vi "Detect Pulses in File.vi"(8 "Delay":dbl=0.013735 format="%#_6p", 9 "Channel name":string="CH0", 10 "I-V parameters":T1={"Start magnitude"=0.01, "Magnitude increment"=0.001, "Number of pulses"=8, "Baseline length"=480, "Ramp length"=32, "Top  length"=480, "Threshold "=1e-05, "Processing delay"=25, "Valhalla range"=0.001, "Interpolation"=64} {"Valhalla range" format="%#_6pA"; "Processing delay" format="%dpts"; "Threshold" format="%#_6pV"; "Top  length" format="%dpts"; "Ramp length" format="%dpts"; "Baseline length" format="%dpts"; "Magnitude increment" format="%#_6pA"; "Start magnitude" format="%#_6pA"}, 11 "File Path":path) -> (0 "Avg signal minus\nAvg background":dbl[](graph), 1 "Pulse indices out":T2[](array[typedef]), 2 "data":waveform(dbl))   [LabVIEW 2016]
uses:
  Pulse indexies.ctl
  I-V parameters.ctl
panel:
  in  "Skip 1st #points":i32=124993
  out "Waveform Graph 2":dbl[][](graph)
  out "Waveform Graph":dbl[][](graph)
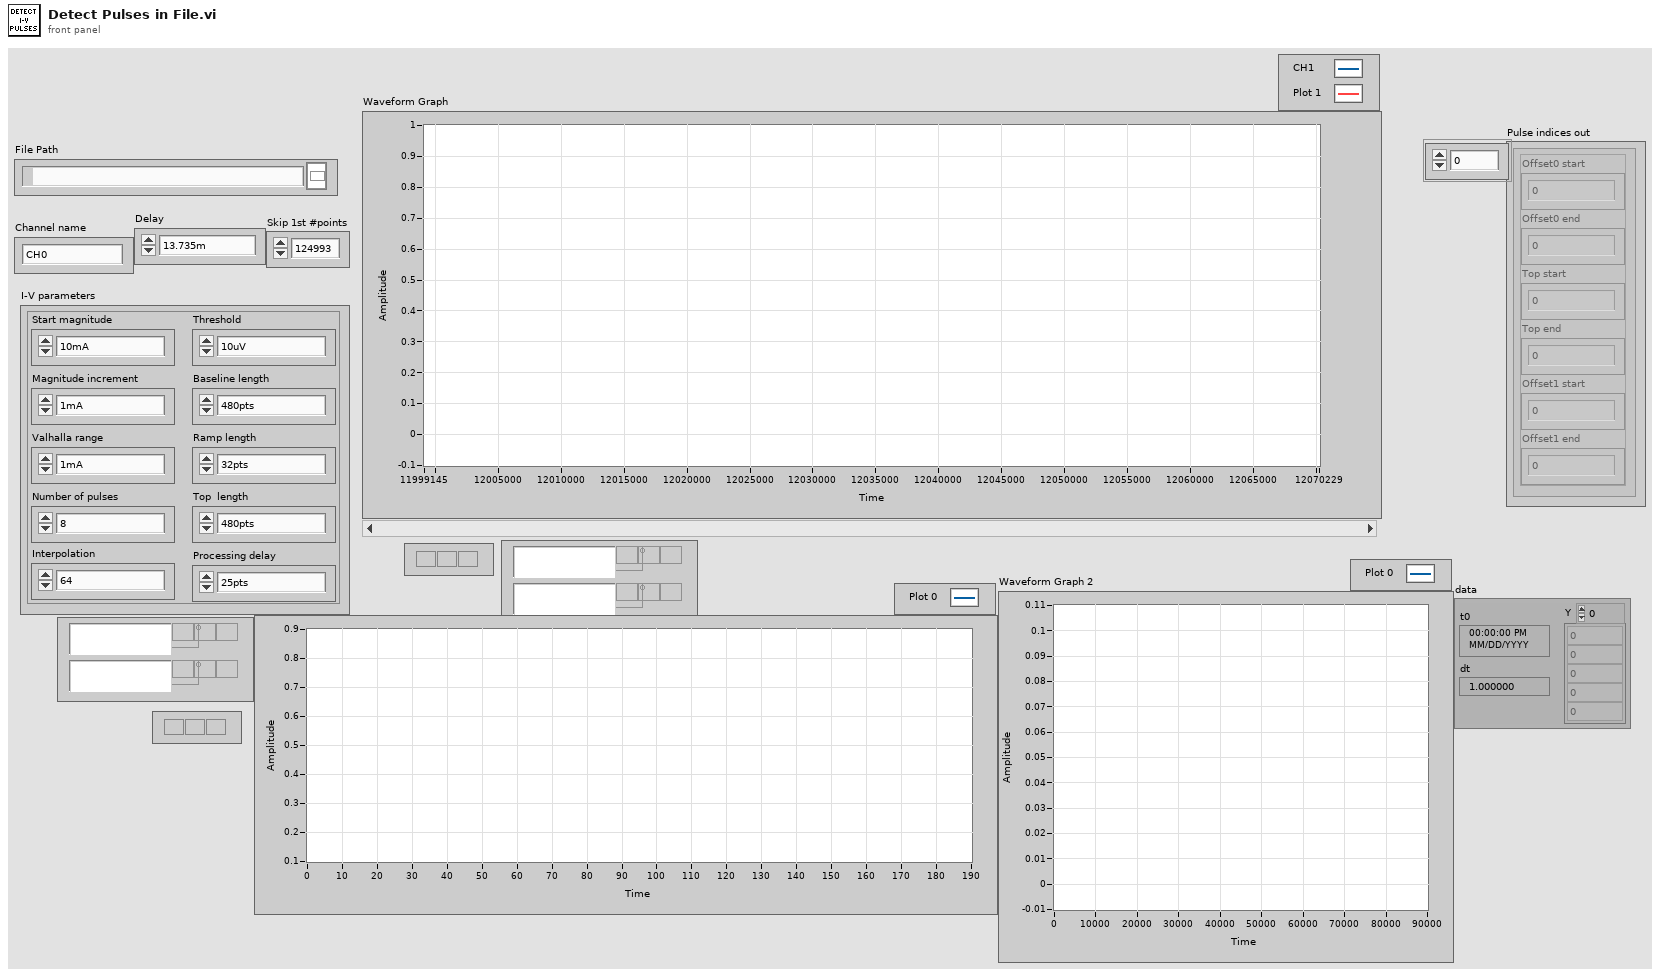
[diagram p1: front panel]
types:
  T1 = typedef "I-V parameters.ctl" = cluster{"Start magnitude":dbl, "Magnitude increment":dbl, "Number of pulses":i32, "Baseline length":i32, "Ramp length":i32, "Top  length":i32, "Threshold ":dbl, "Processing delay":u16, "Valhalla range":dbl, "Interpolation":i32}
  T2 = typedef "Pulse indexies.ctl" = cluster{"Offset0 start ":i32, "Offset0 end":i32, "Top start":i32, "Top end":i32, "Offset1 start":i32, "Offset1 end":i32}
  T3 = enum16{"open", "open or create", "create or replace", "create", "open (read-only)"}
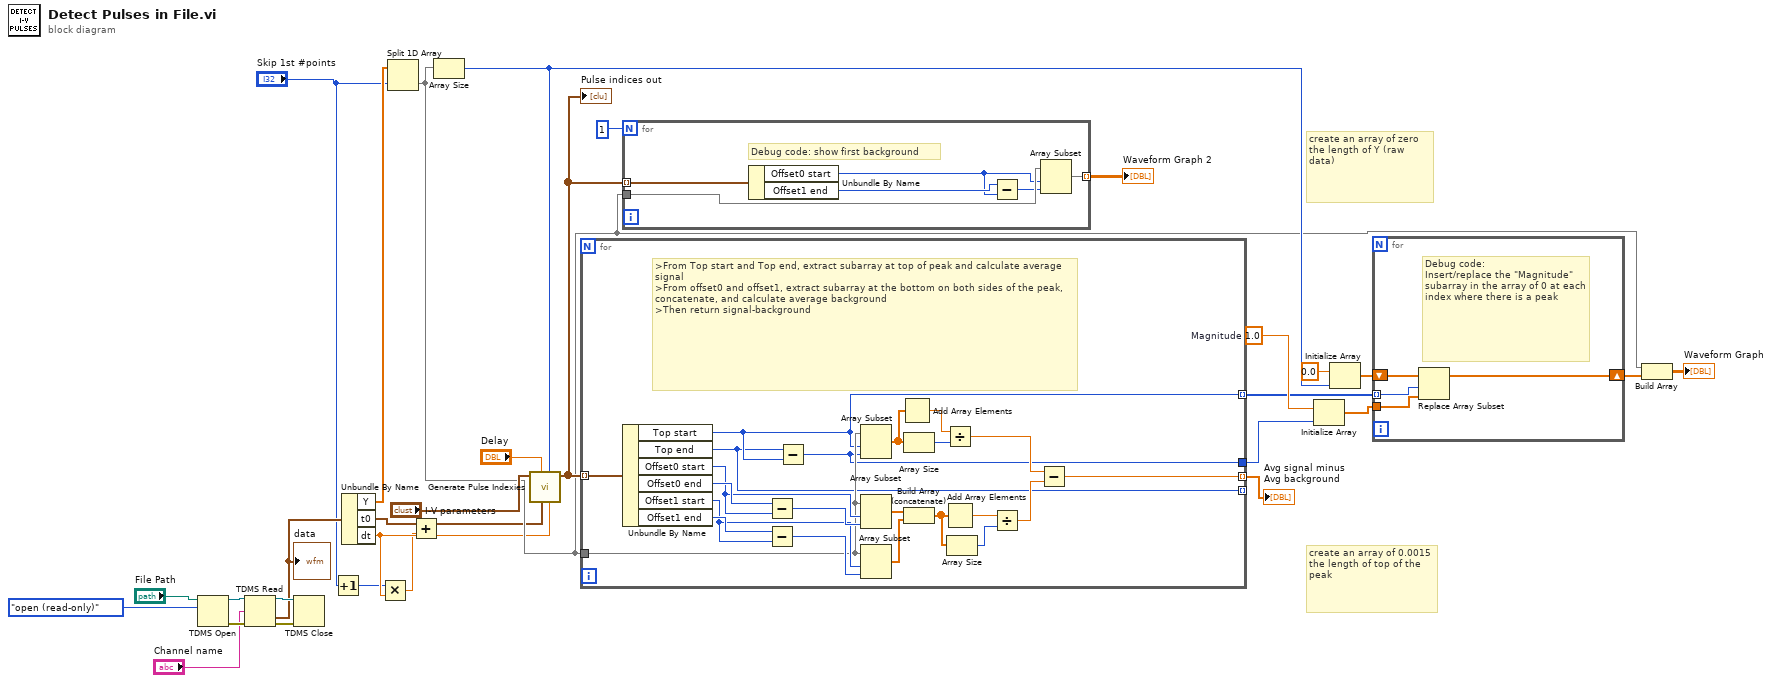
[diagram p0: block diagram]
diagram:
  w14 = 1.0  # Magnitude
  # "create an array of 0.0015 the length of top of the peak"
  # "create an array of zero the length of Y (raw data)"
  n1 = TDMS Open(10:T3."open (read-only)" ("operation (0:open)"), 11:"File Path") -> (0:w29:errorcluster, 3:w31:refnum<k34>)  [unwired: 5 in]
  n2 = TDMS Read(0:w31, 7:"Channel name", 11:w29) -> (4:w30:refnum<k34>, 10:w7:waveform(dbl), 15:w28:errorcluster)  [unwired: 5 in, 3 out]
  "data" <- w7
  n3 = TDMS Close(8:w28, 11:w30) -> ()  [unwired: 2 out]
  n4 = Increment(x="Skip 1st #points") -> (x+1=w1:i32)
  n5 = Unbundle By Name(w7) -> ("Y"=w20:dbl[], "t0"=w24:timestamp, "dt"=w3:dbl)
  n6 = Multiply(x=w1, y=w3) -> (x*y=w2:dbl)
  n7 = Split 1D Array(array=w20, index="Skip 1st #points") -> (second subarray=w6:dbl[])  [unwired: 1 out]
  n8 = Add(x=w24, y=w2) -> (x+y=w5:timestamp)
  n9 = Array Size(array=w6) -> (size(s)=w17:i32)
  n10 = call "Generate Pulse Indexies.vi"("dt"=w3, "Size"=w17, "t0"=w5, "Delay"="Delay", "I-V parameters"="I-V parameters") -> ("Pulse indexies out"=w18:T2[])  [unwired: 6 in]
  "Pulse indices out" <- w18
  n11 = for {
    tunnel: w18 -> [w53] mode=indexing
    tunnel: w6 -> [w46]
    tunnel: [w36] -> w9 mode=indexing
    tunnel: [w34] -> w8 mode=indexing
    tunnel: [w33] -> _ mode=indexing
    tunnel: [w32] -> w15
    # ">From Top start and Top end, extract subarray at top of peak and calculate average signal\n>From offset0 and offset1, extract subarray at the bottom on both sides of the peak, concatenate, and calculate average background\n>Then return signal-background"
    n12 = Unbundle By Name(w53) -> ("Top start"=w34:i32, "Top end"=w33:i32, "Offset0 start"=w51:i32, "Offset0 end"=w52:i32, "Offset1 start"=w48:i32, "Offset1 end"=w49:i32)
    n13 = Subtract(x=w52, y=w51) -> (x-y=w50:i32)
    n14 = Subtract(x=w49, y=w48) -> (x-y=w47:i32)
    n15 = Subtract(x=w33, y=w34) -> (x-y=w32:i32)
    n16 = Array Subset(array=w46, index=w34, length=w32) -> (w43:dbl[])
    n17 = Array Subset(array=w46, index=w51, length=w50) -> (w45:dbl[])
    n18 = Array Subset(array=w46, index=w48, length=w47) -> (w44:dbl[])
    n19 = Add Array Elements(numeric array=w43) -> (sum=w42:dbl)
    n20 = Array Size(array=w43) -> (size(s)=w41:i32)
    n21 = Build Array (concatenate)(w45, w44) -> (w40:dbl[])
    n22 = Divide(x=w42, y=w41) -> (x/y=w37:dbl)
    n23 = Add Array Elements(numeric array=w40) -> (sum=w39:dbl)
    n24 = Array Size(array=w40) -> (size(s)=w38:i32)
    n25 = Divide(x=w39, y=w38) -> (x/y=w35:dbl)
    n26 = Subtract(x=w37, y=w35) -> (x-y=w36:dbl)
  }
  "Avg signal minus\nAvg background" <- w9
  n27 = for {
    N: 1 -> [_]
    tunnel: w18 -> [w58] mode=indexing
    tunnel: w6 -> [w59]
    tunnel: [w54] -> w21 mode=indexing
    # "Debug code: show first background"
    n28 = Unbundle By Name(w58) -> ("Offset0 start"=w56:i32, "Offset1 end"=w57:i32)
    n29 = Subtract(x=w57, y=w56) -> (x-y=w55:i32)
    n30 = Array Subset(array=w59, index=w56, length=w55) -> (w54:dbl[])
  }
  "Waveform Graph 2" <- w21
  n31 = Initialize Array(w14, w15) -> (w13:dbl[])
  n32 = Initialize Array(0.0, w17) -> (w16:dbl[])
  n33 = for {
    tunnel: w8 -> [w62] mode=indexing
    tunnel: w13 -> [w61]
    shift-right: [w60] -> w11
    shift-left: w16 -> [w63]
    # "Debug code:\nInsert/replace the \"Magnitude\" subarray in the array of 0 at each index where there is a peak"
    n34 = Replace Array Subset(array=w63, new element=w61, index=w62) -> (w60:dbl[])
  }
  n35 = Build Array(w6, w11) -> (→"Waveform Graph":dbl[][])
